vi "Autonomous Independent.vi"() -> ()   [LabVIEW 2016]
doc: "This VI is called when autonomous begins, and will automatically be terminated when autonomous ends. You can carry out timed or sensor driven robot movement independently without needing to return to the caller."
uses:
  <vilib>/Rock Robotics/WPI/Solenoid/WPI_SolenoidValue.ctl
  <vilib>/Rock Robotics/WPI/ThirdParty/Sensors/navX/_TypeDefs/FRIC_navX_DeviceNumbersTypeDef.ctl
  <vilib>/Rock Robotics/WPI/Utilities/WPI_GetSetVariantRefNum.vi
  <vilib>/Rock Robotics/Network Tables/NT Read String.vi
  <vilib>/Rock Robotics/WPI/Solenoid/WPI_SolenoidSetEnum.vi
  <vilib>/Rock Robotics/Network Tables/NT Write Number.vi
  <vilib>/addons/control/pid/pid.llb/PID (DBL).vi
  <vilib>/Rock Robotics/Network Tables/NT Write Numeric Array.vi
  <vilib>/addons/control/pid/NI_PID_pid.lvlib
panel:
  out "Distance 11":dbl
  out "Distance 10":dbl
  out "Distance 9":dbl
  out "Distance 8":dbl
  out "Distance 7":dbl
  out "Distance 6":dbl
  out "Distance 5":dbl
  out "Distance 4":dbl
  out "Distance 3":dbl
  out "Distance 2":dbl
  out "Distance 0":dbl
  out "Distance 1":dbl
  # "Be sure to right-click and choose Data Operations>>Make Current Value default if you want to save the array values with the VI"
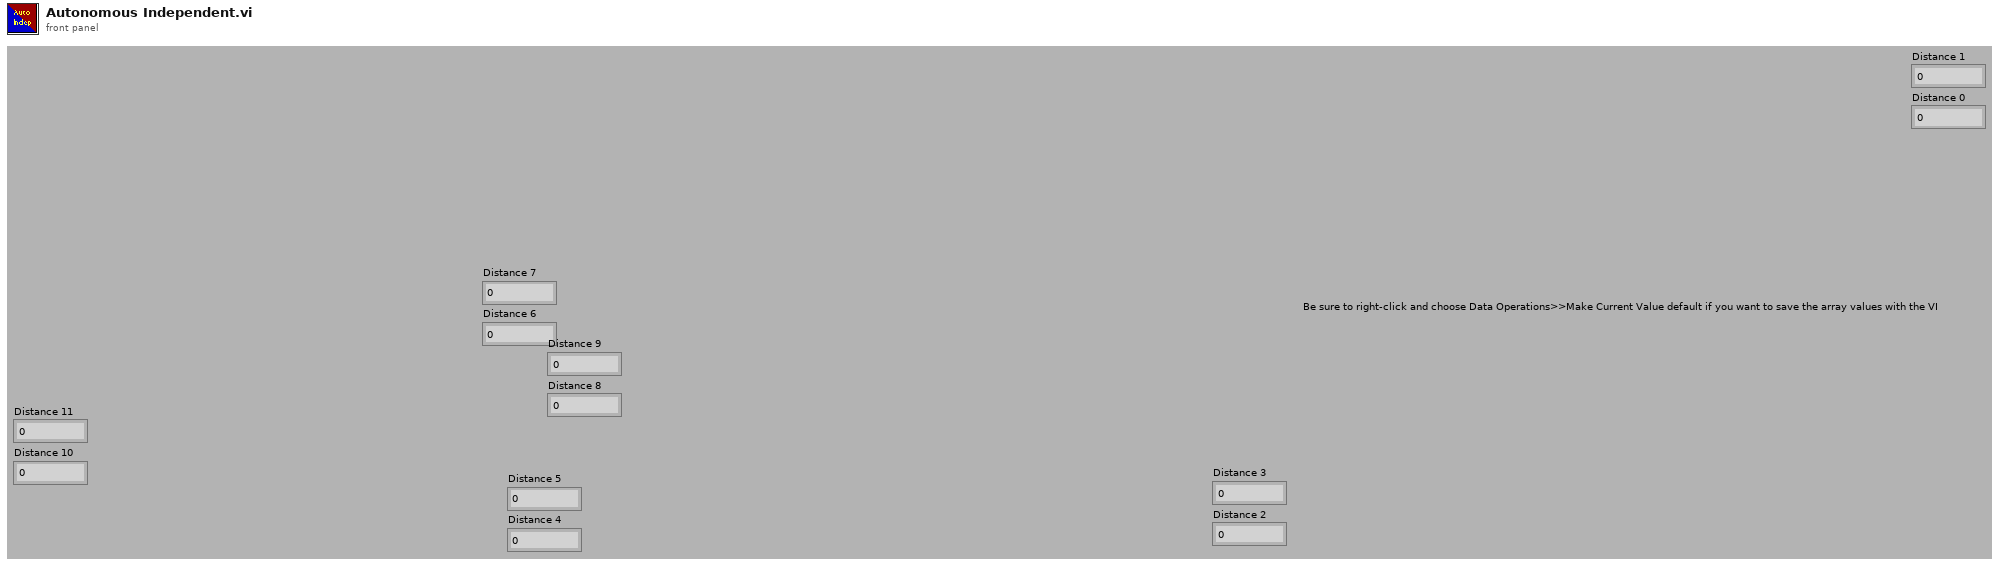
[diagram p1: front panel]
types:
  T1 = typedef "WPI_JoystickDevRef.ctl" = cluster{"Device":T2}
  T2 = typedef "WPI_JoystickDeviceEnum.ctl" = enum16{"USB 0", "USB 1", "USB 2", "USB 3", "USB 4", "USB 5"}
  T3 = typedef "WPI_SolenoidValue.ctl" = enum16{"Off", "On", "Forward", "Reverse"}
  T4 = typedef "FRIC_navX_DeviceNumbersTypeDef.ctl" = enum16{"Dev0", "Dev1", "Dev2", "Dev3"}
  T5 = cluster{"proportional gain (Kc)":dbl, "integral time (Ti, min)":dbl, "derivative time (Td, min)":dbl}
  T6 = typedef "WPI_SolenoidDevRef.ctl" = cluster{"DevStatus":errorcluster, "Pneumatics Control Module":u8, "Forward Solenoid Channel":T7, "Reverse Solenoid Channel":T7}
  T7 = typedef "WPI_SolenoidChannel.ctl" = enum8{"Solenoid 0", "Solenoid 1", "Solenoid 2", "Solenoid 3", "Solenoid 4", "Solenoid 5", "Solenoid 6", "Solenoid 7", "Invalid"}
  T8 = typedef "WPI_RobotDriveDevRef.ctl" = cluster{"DevStatus":errorcluster, "Motors[]":T9[], "Square Inputs":bool, "Max Output":dbl}
  T9 = typedef "WPI_MotorControlDeviceRef.ctl" = cluster{"DeviceStatus":errorcluster, "Type":T10, "PWM":cluster{"PWM Channel":T11, "DeadBand":T12}, "CAN":cluster{"Device Number":u8, "SetOutput VI Ref":variant, "GetOutput VI Ref":variant, "Enable VI Ref":variant, "Disable VI Ref":variant, "Data":variant}, "Invert":bool}
  T10 = typedef "WPI_MotorControlType.ctl" = enum16{"PWM", "CAN"}
  T11 = typedef "FPGA_DIOPWMChannel.ctl" = enum8{"PWM 0", "PWM 1", "PWM 2", "PWM 3", "PWM 4", "PWM 5", "PWM 6", "PWM 7", "PWM 8", "PWM 9", "PWM MXP 0", "PWM MXP 1", "PWM MXP 2", "PWM MXP 3", "PWM MXP 4", "PWM MXP 5", "PWM MXP 6", "PWM MXP 7", "PWM MXP 8", "PWM MXP 9", "Invalid"}
  T12 = typedef "WPI_PWMDeadband.ctl" = cluster{"Name":string, "maxPositivePwm":i32, "minPositivePwm":i32, "centerPwm":i32, "maxNegativePwm":i32, "minNegativePwm":i32, "angularRange":u16}
  T13 = typedef "WPI_EncoderDevRef.ctl" = cluster{"DevStatus":errorcluster, "EncoderIndex":T14, "CounterIndex":T15, "DistancePerCount":dbl, "Decoding Type":T16}
  T14 = typedef "FPGA_EncoderIdx.ctl" = enum8{"Enc 0", "Enc 1", "Enc 2", "Enc 3", "Enc 4", "Enc 5", "Enc 6", "Enc 7", "Invalid"}
  T15 = typedef "FPGA_CounterCtrSystemIndex.ctl" = enum8{"Ctr 0", "Ctr 1", "Ctr 2", "Ctr 3", "Ctr 4", "Ctr 5", "Ctr 6", "Ctr 7", "Invalid"}
  T16 = typedef "WPI_EncoderType.ctl" = enum16{"1x", "2x", "4x"}
  T17 = cluster{"Yaw":dbl, "Roll":dbl, "Pitch":dbl, "Heading":dbl, "Fused Heading":dbl}
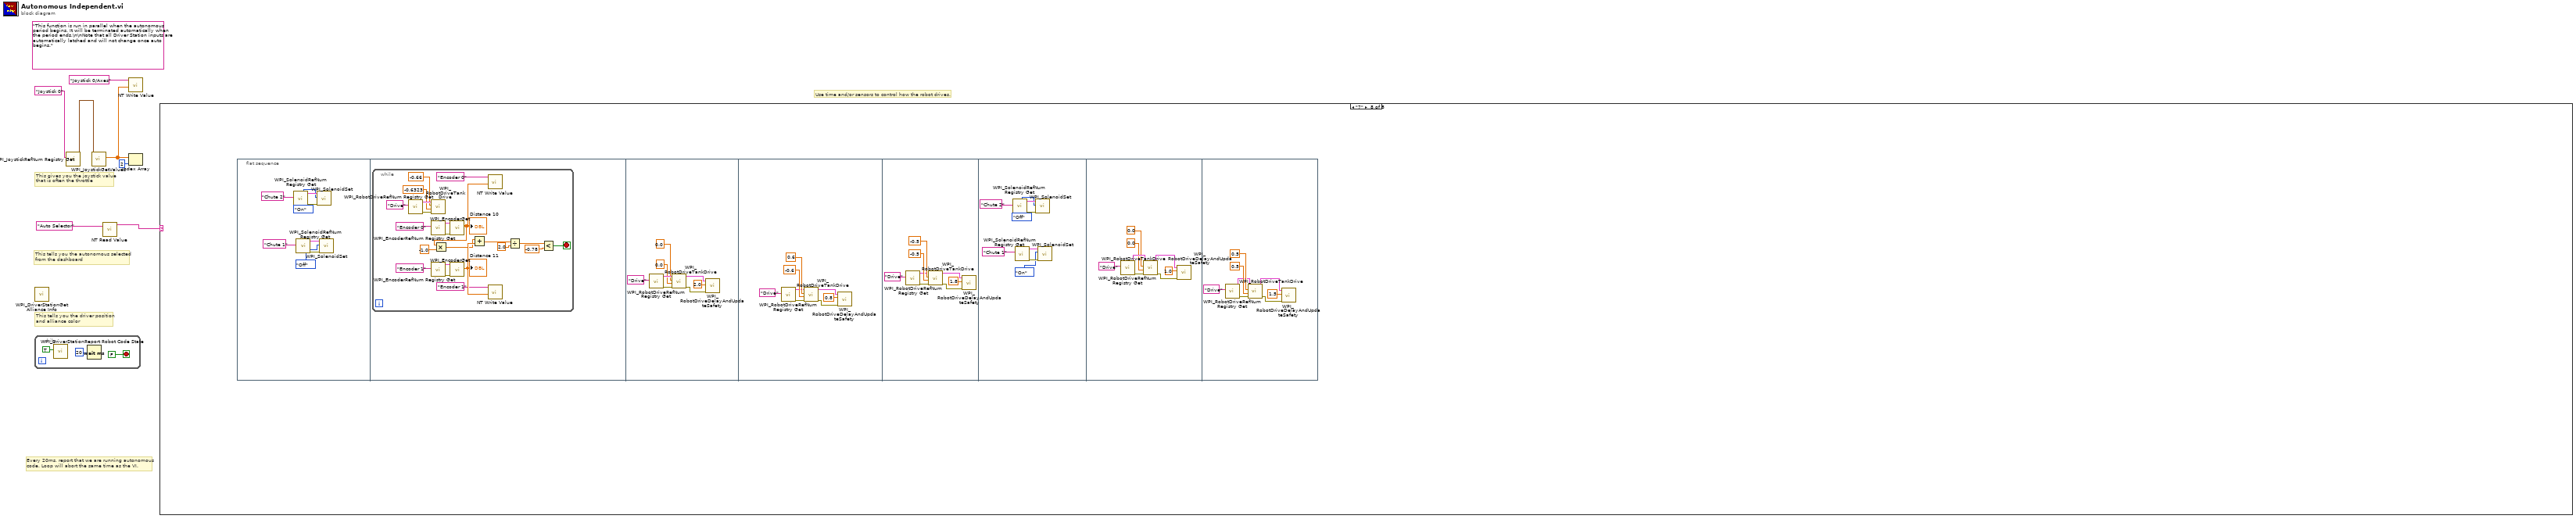
[diagram p0: block diagram]
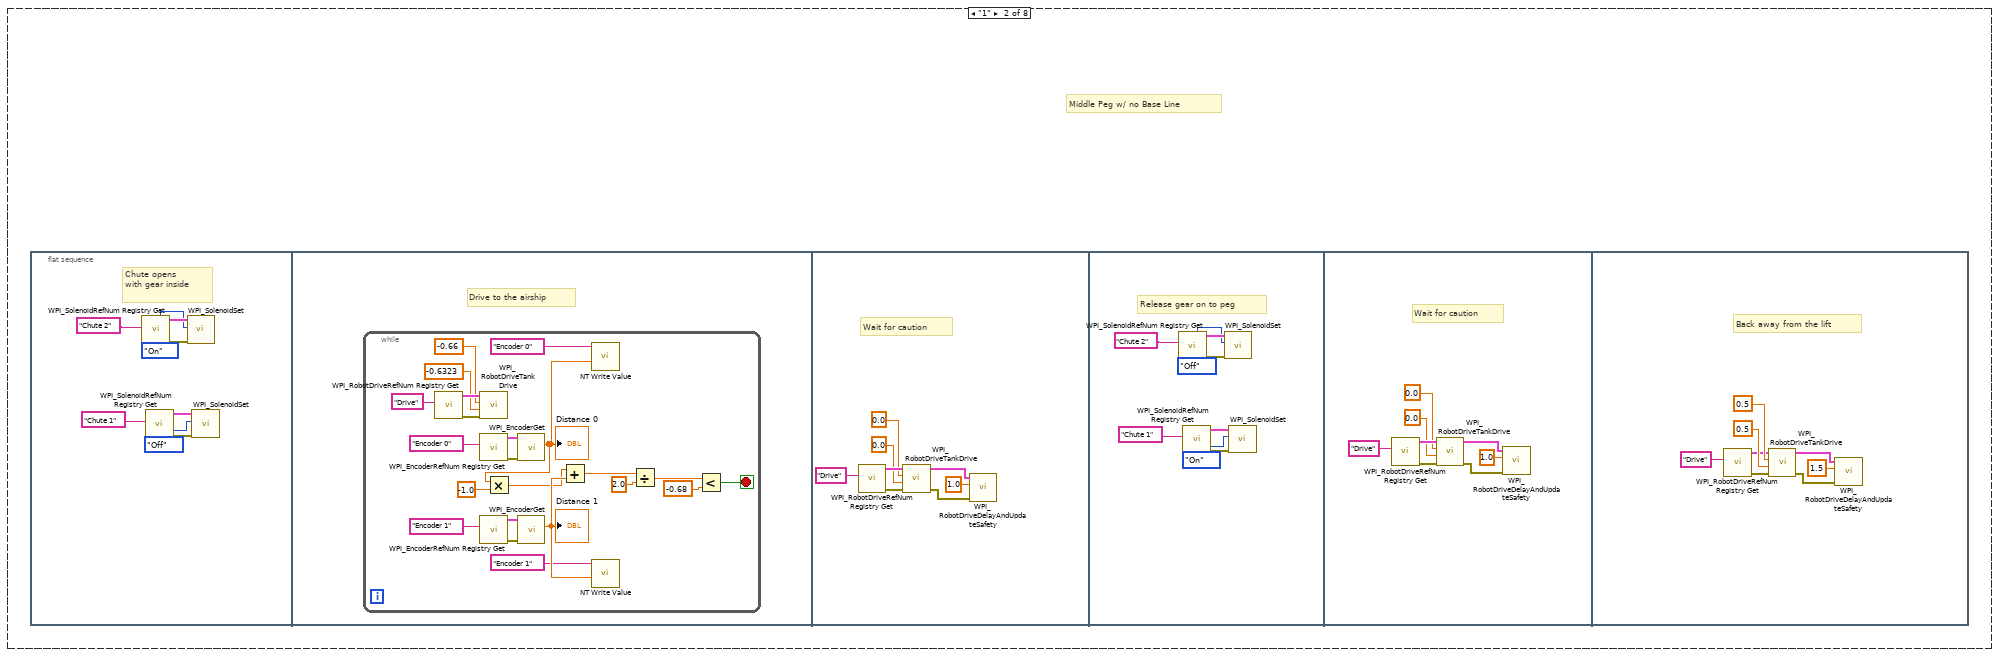
[diagram p3: hidden frame]
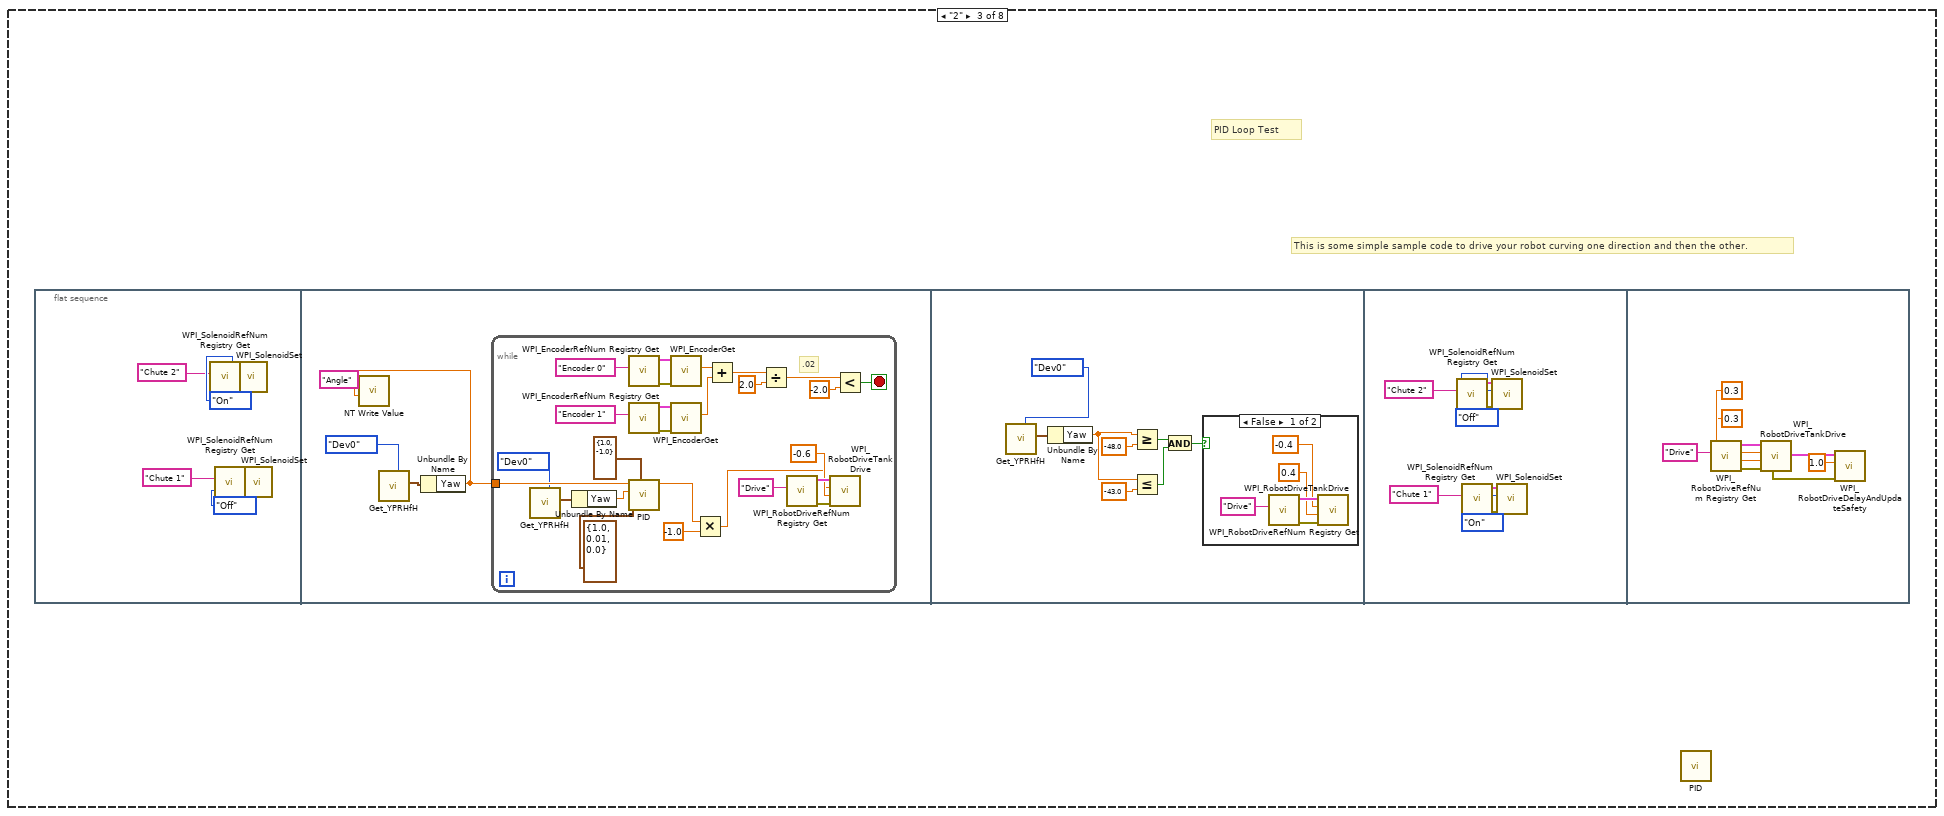
[diagram p4: hidden frame]
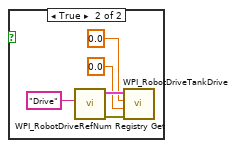
[diagram p5: hidden frame]
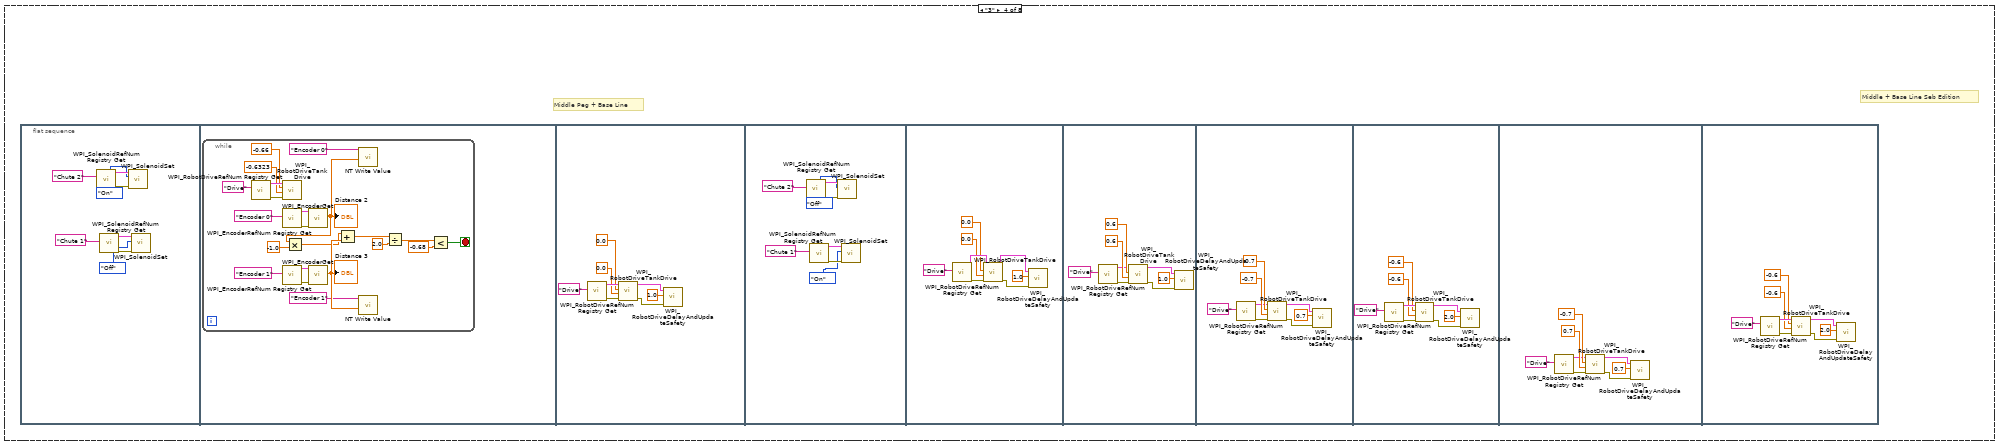
[diagram p6: hidden frame]
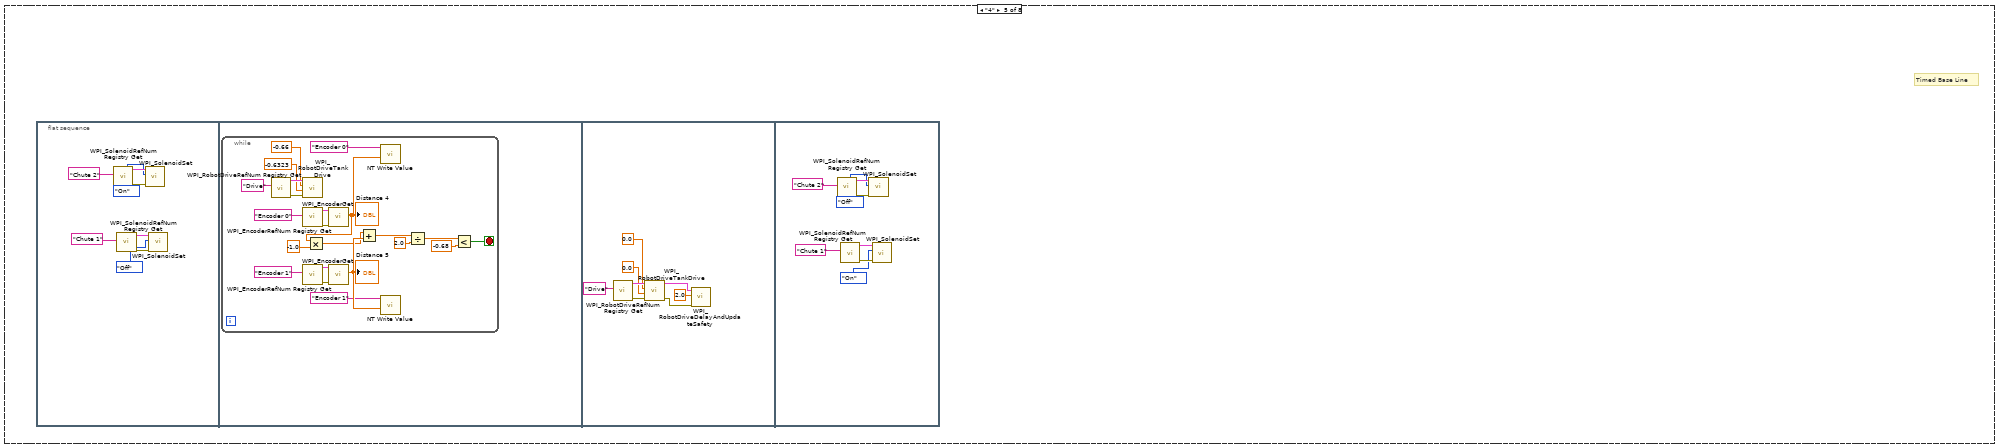
[diagram p7: hidden frame]
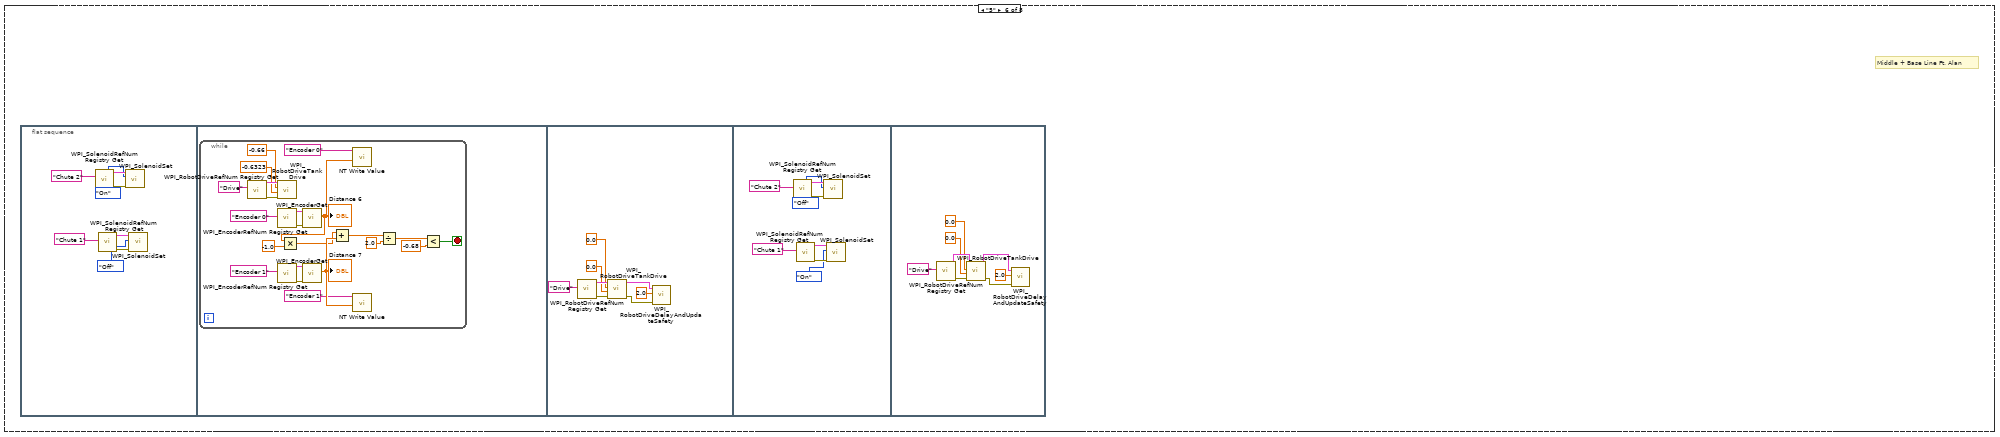
[diagram p8: hidden frame]
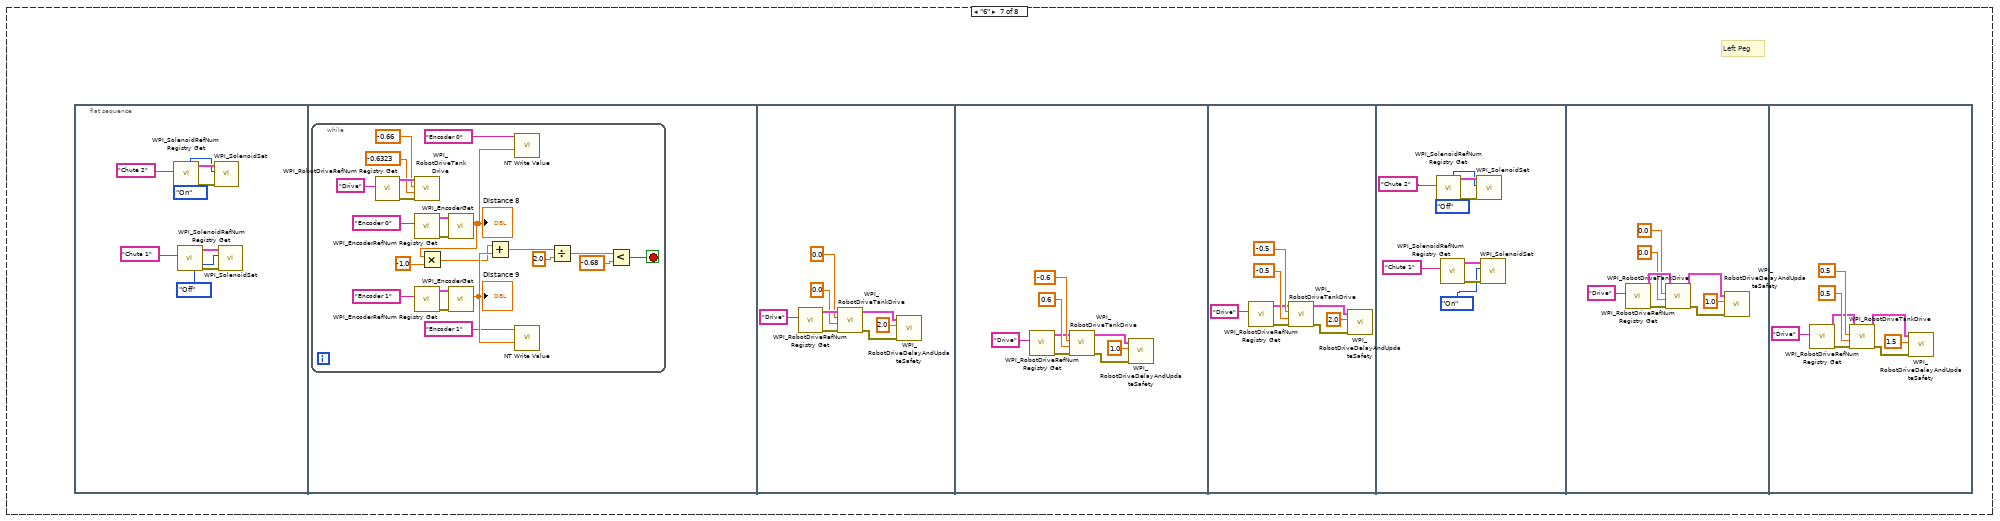
[diagram p9: hidden frame]
diagram:
  (unwired) "This function is run in parallel when the autonomous period begins. It will be terminated automatically when the period ends.\n\nNote that all Driver Station inputs are automatically latched and will not change once auto begins."
  # "This tells you the autonomous selected\nfrom the dashboard"
  # "Every 20ms, report that we are running autonomous\ncode. Loop will abort the same time as the VI."
  # "This gives you the joystick value\nthat is often the throttle"
  # "Use time and/or sensors to control how the robot drives."
  # "This tells you the driver position\nand alliance color"
  n1 = while {
    stop <- FALSE stop-if-true
    n2 = call <vilib>:"WPI_DriverStationReport Robot Code State.vi"("Autonomous"=TRUE) -> ()  [unwired: 10 in, 1 out]
    n3 = Wait (ms)(milliseconds to wait=u32 20) -> ()  [unwired: 1 out]
  }
  n4 = call <vilib>:"WPI_DriverStationGet Alliance Info.vi"() -> ()  [unwired: 12 out]
  n5 = call <vilib>:"WPI_JoystickRefNum Registry Get.vi"("refnum name"="Joystick 0") -> ("JoystickDevRef"=w6:T1)  [unwired: 1 in, 9 out]
  n6 = call <vilib>:"WPI_JoystickGetValues.vi"("JoystickDevRef"=w6) -> ("Axes"=w2:dbl[])  [unwired: 6 in, 4 out]
  n7 = call-poly <vilib>:"NT Read Value.vi"("Name"="Auto Selector") -> ("String"=w3:string)  [unwired: 9 in, 1 out]
  n8 = call-poly <vilib>:"NT Write Value.vi"("Numeric Array"=w2, "Name"="Joystick 0/Axes") -> ()  [unwired: 9 in, 1 out]
  n9 = Index Array(array=w2, index=2) -> ()  [unwired: 1 out]
  n10 = case shown="\"7\"" w3 {
    frame Default {
    }
    frame "1" {
      # "Middle Peg w/ no Base Line"
      n11 = flat-sequence {
        frame #0 {
          # "Chute opens\nwith gear inside"
          n12 = call <vilib>:"WPI_SolenoidRefNum Registry Get.vi"("refnum name"="Chute 2") -> ("error out"=w18:errorcluster, "SolenoidDevRef"=w17:T6)  [unwired: 9 in]
          n13 = call <vilib>:"WPI_SolenoidRefNum Registry Get.vi"("refnum name"="Chute 1") -> ("error out"=w14:errorcluster, "SolenoidDevRef"=w13:T6)  [unwired: 9 in]
          n14 = call-poly <vilib>:"WPI_SolenoidSet.vi"("error in (no error)"=w18, "Value"=WPI_SolenoidValue."On", "SolenoidDevRef"=w17) -> ()  [unwired: 7 in, 2 out]
          n15 = call-poly <vilib>:"WPI_SolenoidSet.vi"("error in (no error)"=w14, "Value"=WPI_SolenoidValue."Off", "SolenoidDevRef"=w13) -> ()  [unwired: 7 in, 2 out]
        }
        frame #1 {
          # "Drive to the airship"
          n16 = while {
            stop <- w26 stop-if-true
            n17 = call <vilib>:"WPI_RobotDriveRefNum Registry Get.vi"("refnum name"="Drive") -> ("error out"=w39:errorcluster, "RobotDriveDevRef"=w40:T8)  [unwired: 9 in]
            n18 = call <vilib>:"WPI_RobotDriveTankDrive.vi"("error in (no error)"=w39, "Right axis value"=-0.6323, "Left axis value"=-0.66, "RobotDriveDevRef"=w40) -> ()  [unwired: 5 in, 3 out]
            n19 = call <vilib>:"WPI_EncoderRefNum Registry Get.vi"("refnum name"="Encoder 0") -> ("error out"=w35:errorcluster, "EncoderDevRef"=w34:T13)  [unwired: 9 in]
            n20 = call <vilib>:"WPI_EncoderRefNum Registry Get.vi"("refnum name"="Encoder 1") -> ("error out"=w32:errorcluster, "EncoderDevRef"=w31:T13)  [unwired: 9 in]
            n21 = call <vilib>:"WPI_EncoderGet.vi"("error in (no error)"=w35, "EncoderDevRef"=w34) -> ("Distance"=w20:dbl)  [unwired: 4 in, 5 out]
            "Distance 0" <- w20
            n22 = Multiply(x=w20, y=-1.0) -> (x*y=w19:dbl)
            n23 = call <vilib>:"WPI_EncoderGet.vi"("error in (no error)"=w32, "EncoderDevRef"=w31) -> ("Distance"=w23:dbl)  [unwired: 4 in, 5 out]
            "Distance 1" <- w23
            n24 = Add(x=w19, y=w23) -> (x+y=w29:dbl)
            n25 = call-poly <vilib>:"NT Write Value.vi"("Numeric"=w20, "Name"="Encoder 0") -> ()  [unwired: 9 in, 1 out]
            n26 = call-poly <vilib>:"NT Write Value.vi"("Numeric"=w23, "Name"="Encoder 1") -> ()  [unwired: 9 in, 1 out]
            n27 = Divide(x=w29, y=2.0) -> (x/y=w27:dbl)
            n28 = Less?(x=w27, y=-0.68) -> (x < y?=w26:bool)
          }
        }
        frame #2 {
          # "Wait for caution"
          n29 = call <vilib>:"WPI_RobotDriveRefNum Registry Get.vi"("refnum name"="Drive") -> ("error out"=w44:errorcluster, "RobotDriveDevRef"=w45:T8)  [unwired: 9 in]
          n30 = call <vilib>:"WPI_RobotDriveTankDrive.vi"("error in (no error)"=w44, "Right axis value"=0.0, "Left axis value"=0.0, "RobotDriveDevRef"=w45) -> ("error out"=w47:errorcluster, "RobotDriveDevRef"=w46:T8)  [unwired: 5 in, 1 out]
          n31 = call <vilib>:"WPI_RobotDriveDelayAndUpdateSafety.vi"("error in (no error)"=w47, "Delay (s)"=1.0, "RobotDriveDevRef"=w46) -> ()  [unwired: 7 in, 2 out]
        }
        frame #3 {
          # "Release gear on to peg"
          n32 = call <vilib>:"WPI_SolenoidRefNum Registry Get.vi"("refnum name"="Chute 2") -> ("error out"=w56:errorcluster, "SolenoidDevRef"=w55:T6)  [unwired: 9 in]
          n33 = call <vilib>:"WPI_SolenoidRefNum Registry Get.vi"("refnum name"="Chute 1") -> ("error out"=w52:errorcluster, "SolenoidDevRef"=w51:T6)  [unwired: 9 in]
          n34 = call-poly <vilib>:"WPI_SolenoidSet.vi"("error in (no error)"=w56, "Value"=WPI_SolenoidValue."Off", "SolenoidDevRef"=w55) -> ()  [unwired: 7 in, 2 out]
          n35 = call-poly <vilib>:"WPI_SolenoidSet.vi"("error in (no error)"=w52, "Value"=WPI_SolenoidValue."On", "SolenoidDevRef"=w51) -> ()  [unwired: 7 in, 2 out]
        }
        frame #4 {
          # "Wait for caution"
          n36 = call <vilib>:"WPI_RobotDriveRefNum Registry Get.vi"("refnum name"="Drive") -> ("error out"=w60:errorcluster, "RobotDriveDevRef"=w61:T8)  [unwired: 9 in]
          n37 = call <vilib>:"WPI_RobotDriveTankDrive.vi"("error in (no error)"=w60, "Right axis value"=0.0, "Left axis value"=0.0, "RobotDriveDevRef"=w61) -> ("error out"=w63:errorcluster, "RobotDriveDevRef"=w62:T8)  [unwired: 5 in, 1 out]
          n38 = call <vilib>:"WPI_RobotDriveDelayAndUpdateSafety.vi"("error in (no error)"=w63, "Delay (s)"=1.0, "RobotDriveDevRef"=w62) -> ()  [unwired: 7 in, 2 out]
        }
        frame #5 {
          # "Back away from the lift"
          n39 = call <vilib>:"WPI_RobotDriveRefNum Registry Get.vi"("refnum name"="Drive") -> ("error out"=w69:errorcluster, "RobotDriveDevRef"=w68:T8)  [unwired: 9 in]
          n40 = call <vilib>:"WPI_RobotDriveTankDrive.vi"("error in (no error)"=w69, "Right axis value"=0.5, "Left axis value"=0.5, "RobotDriveDevRef"=w68) -> ("error out"=w66:errorcluster, "RobotDriveDevRef"=w67:T8)  [unwired: 5 in, 1 out]
          n41 = call <vilib>:"WPI_RobotDriveDelayAndUpdateSafety.vi"("error in (no error)"=w66, "Delay (s)"=1.5, "RobotDriveDevRef"=w67) -> ()  [unwired: 7 in, 2 out]
        }
      }
    }
    frame "2" {
      # "PID Loop Test"
      # "This is some simple sample code to drive your robot curving one direction and then the other."
      n42 = flat-sequence {
        frame #0 {
          n43 = call <vilib>:"WPI_SolenoidRefNum Registry Get.vi"("refnum name"="Chute 2") -> ("error out"=w80:errorcluster, "SolenoidDevRef"=w79:T6)  [unwired: 9 in]
          n44 = call <vilib>:"WPI_SolenoidRefNum Registry Get.vi"("refnum name"="Chute 1") -> ("error out"=w76:errorcluster, "SolenoidDevRef"=w75:T6)  [unwired: 9 in]
          n45 = call-poly <vilib>:"WPI_SolenoidSet.vi"("error in (no error)"=w80, "Value"=WPI_SolenoidValue."On", "SolenoidDevRef"=w79) -> ()  [unwired: 7 in, 2 out]
          n46 = call-poly <vilib>:"WPI_SolenoidSet.vi"("error in (no error)"=w76, "Value"=WPI_SolenoidValue."Off", "SolenoidDevRef"=w75) -> ()  [unwired: 7 in, 2 out]
        }
        frame #1 {
          n47 = call <vilib>:"Get_YPRHfH.vi"("Device Number"=FRIC_navX_DeviceNumbersTypeDef."Dev0") -> ("YRPHfH"=w84:T17)  [unwired: 10 in]
          n48 = Unbundle By Name(w84) -> ("Yaw"=w83:dbl)
          n49 = call-poly <vilib>:"NT Write Value.vi"("Numeric"=w83, "Name"="Angle") -> ()  [unwired: 9 in, 1 out]
          n50 = while {
            tunnel: w83 -> [w96]
            stop <- w99 stop-if-true
            # ".02"
            n51 = call <vilib>:"Get_YPRHfH.vi"("Device Number"=FRIC_navX_DeviceNumbersTypeDef."Dev0") -> ("YRPHfH"=w97:T17)  [unwired: 10 in]
            n52 = Unbundle By Name(w97) -> ("Yaw"=w95:dbl)
            n53 = call <vilib>:"WPI_EncoderRefNum Registry Get.vi"("refnum name"="Encoder 0") -> ("error out"=w110:errorcluster, "EncoderDevRef"=w109:T13)  [unwired: 9 in]
            n54 = call <vilib>:"WPI_EncoderRefNum Registry Get.vi"("refnum name"="Encoder 1") -> ("error out"=w107:errorcluster, "EncoderDevRef"=w106:T13)  [unwired: 9 in]
            n55 = call-poly <vilib>:"PID.vi"("output range"=cluster{"output high":dbl, "output low":dbl} {"output high"=1.0, "output low"=-1.0}, "PID gains"=T5 {"proportional gain (Kc)"=1.0, "integral time (Ti, min)"=0.01, "derivative time (Td, min)"=0.0}, "process variable"=w95, "setpoint"=w96) -> ("output"=w87:dbl)  [unwired: 6 in, 1 out]
            n56 = call <vilib>:"WPI_EncoderGet.vi"("error in (no error)"=w110, "EncoderDevRef"=w109) -> ("Distance"=w103:dbl)  [unwired: 4 in, 5 out]
            n57 = call <vilib>:"WPI_EncoderGet.vi"("error in (no error)"=w107, "EncoderDevRef"=w106) -> ("Distance"=w104:dbl)  [unwired: 4 in, 5 out]
            n58 = Multiply(x=w87, y=-1.0) -> (x*y=w86:dbl)
            n59 = Add(x=w103, y=w104) -> (x+y=w102:dbl)
            n60 = Divide(x=w102, y=2.0) -> (x/y=w100:dbl)
            n61 = call <vilib>:"WPI_RobotDriveRefNum Registry Get.vi"("refnum name"="Drive") -> ("error out"=w91:errorcluster, "RobotDriveDevRef"=w92:T8)  [unwired: 9 in]
            n62 = call <vilib>:"WPI_RobotDriveTankDrive.vi"("error in (no error)"=w91, "Right axis value"=-0.6, "Left axis value"=w86, "RobotDriveDevRef"=w92) -> ()  [unwired: 5 in, 3 out]
            n63 = Less?(x=w100, y=-2.0) -> (x < y?=w99:bool)
          }
        }
        frame #2 {
          n64 = call <vilib>:"Get_YPRHfH.vi"("Device Number"=FRIC_navX_DeviceNumbersTypeDef."Dev0") -> ("YRPHfH"=w118:T17)  [unwired: 10 in]
          n65 = Unbundle By Name(w118) -> ("Yaw"=w113:dbl)
          n66 = Greater Or Equal?(x=w113, y=-48.0) -> (x >= y?=w116:bool)
          n67 = Less Or Equal?(x=w113, y=-43.0) -> (x <= y?=w115:bool)
          n68 = And(x=w116, y=w115) -> (x .and. y?=w112:bool)
          n69 = case shown="False" w112 {
            frame False {
              n70 = call <vilib>:"WPI_RobotDriveRefNum Registry Get.vi"("refnum name"="Drive") -> ("error out"=w122:errorcluster, "RobotDriveDevRef"=w123:T8)  [unwired: 9 in]
              n71 = call <vilib>:"WPI_RobotDriveTankDrive.vi"("error in (no error)"=w122, "Right axis value"=0.4, "Left axis value"=-0.4, "RobotDriveDevRef"=w123) -> ()  [unwired: 5 in, 3 out]
            }
            frame True {
              n72 = call <vilib>:"WPI_RobotDriveRefNum Registry Get.vi"("refnum name"="Drive") -> ("error out"=w127:errorcluster, "RobotDriveDevRef"=w128:T8)  [unwired: 9 in]
              n73 = call <vilib>:"WPI_RobotDriveTankDrive.vi"("error in (no error)"=w127, "Right axis value"=0.0, "Left axis value"=0.0, "RobotDriveDevRef"=w128) -> ()  [unwired: 5 in, 3 out]
            }
          }
        }
        frame #3 {
          n74 = call <vilib>:"WPI_SolenoidRefNum Registry Get.vi"("refnum name"="Chute 2") -> ("error out"=w136:errorcluster, "SolenoidDevRef"=w135:T6)  [unwired: 9 in]
          n75 = call <vilib>:"WPI_SolenoidRefNum Registry Get.vi"("refnum name"="Chute 1") -> ("error out"=w132:errorcluster, "SolenoidDevRef"=w131:T6)  [unwired: 9 in]
          n76 = call-poly <vilib>:"WPI_SolenoidSet.vi"("error in (no error)"=w136, "Value"=WPI_SolenoidValue."Off", "SolenoidDevRef"=w135) -> ()  [unwired: 7 in, 2 out]
          n77 = call-poly <vilib>:"WPI_SolenoidSet.vi"("error in (no error)"=w132, "Value"=WPI_SolenoidValue."On", "SolenoidDevRef"=w131) -> ()  [unwired: 7 in, 2 out]
        }
        frame #4 {
          n78 = call <vilib>:"WPI_RobotDriveRefNum Registry Get.vi"("refnum name"="Drive") -> ("error out"=w141:errorcluster, "RobotDriveDevRef"=w140:T8)  [unwired: 9 in]
          n79 = call <vilib>:"WPI_RobotDriveTankDrive.vi"("error in (no error)"=w141, "Right axis value"=0.3, "Left axis value"=0.3, "RobotDriveDevRef"=w140) -> ("error out"=w138:errorcluster, "RobotDriveDevRef"=w139:T8)  [unwired: 5 in, 1 out]
          n80 = call <vilib>:"WPI_RobotDriveDelayAndUpdateSafety.vi"("error in (no error)"=w138, "Delay (s)"=1.0, "RobotDriveDevRef"=w139) -> ()  [unwired: 7 in, 2 out]
        }
      }
      n81 = call-poly <vilib>:"PID.vi"() -> ()  [unwired: 10 in, 2 out]
    }
    frame "3" {
      # "Middle + Base Line Seb Edition"
      # "Middle Peg + Base Line"
      n82 = flat-sequence {
        frame #0 {
          n83 = call <vilib>:"WPI_SolenoidRefNum Registry Get.vi"("refnum name"="Chute 2") -> ("error out"=w152:errorcluster, "SolenoidDevRef"=w151:T6)  [unwired: 9 in]
          n84 = call <vilib>:"WPI_SolenoidRefNum Registry Get.vi"("refnum name"="Chute 1") -> ("error out"=w148:errorcluster, "SolenoidDevRef"=w147:T6)  [unwired: 9 in]
          n85 = call-poly <vilib>:"WPI_SolenoidSet.vi"("error in (no error)"=w152, "Value"=WPI_SolenoidValue."On", "SolenoidDevRef"=w151) -> ()  [unwired: 7 in, 2 out]
          n86 = call-poly <vilib>:"WPI_SolenoidSet.vi"("error in (no error)"=w148, "Value"=WPI_SolenoidValue."Off", "SolenoidDevRef"=w147) -> ()  [unwired: 7 in, 2 out]
        }
        frame #1 {
          n87 = while {
            stop <- w160 stop-if-true
            n88 = call <vilib>:"WPI_RobotDriveRefNum Registry Get.vi"("refnum name"="Drive") -> ("error out"=w173:errorcluster, "RobotDriveDevRef"=w174:T8)  [unwired: 9 in]
            n89 = call <vilib>:"WPI_RobotDriveTankDrive.vi"("error in (no error)"=w173, "Right axis value"=-0.6323, "Left axis value"=-0.66, "RobotDriveDevRef"=w174) -> ()  [unwired: 5 in, 3 out]
            n90 = call <vilib>:"WPI_EncoderRefNum Registry Get.vi"("refnum name"="Encoder 0") -> ("error out"=w169:errorcluster, "EncoderDevRef"=w168:T13)  [unwired: 9 in]
            n91 = call <vilib>:"WPI_EncoderRefNum Registry Get.vi"("refnum name"="Encoder 1") -> ("error out"=w166:errorcluster, "EncoderDevRef"=w165:T13)  [unwired: 9 in]
            n92 = call <vilib>:"WPI_EncoderGet.vi"("error in (no error)"=w169, "EncoderDevRef"=w168) -> ("Distance"=w154:dbl)  [unwired: 4 in, 5 out]
            "Distance 2" <- w154
            n93 = Multiply(x=w154, y=-1.0) -> (x*y=w153:dbl)
            n94 = call <vilib>:"WPI_EncoderGet.vi"("error in (no error)"=w166, "EncoderDevRef"=w165) -> ("Distance"=w157:dbl)  [unwired: 4 in, 5 out]
            "Distance 3" <- w157
            n95 = Add(x=w153, y=w157) -> (x+y=w163:dbl)
            n96 = call-poly <vilib>:"NT Write Value.vi"("Numeric"=w154, "Name"="Encoder 0") -> ()  [unwired: 9 in, 1 out]
            n97 = call-poly <vilib>:"NT Write Value.vi"("Numeric"=w157, "Name"="Encoder 1") -> ()  [unwired: 9 in, 1 out]
            n98 = Divide(x=w163, y=2.0) -> (x/y=w161:dbl)
            n99 = Less?(x=w161, y=-0.68) -> (x < y?=w160:bool)
          }
        }
        frame #2 {
          n100 = call <vilib>:"WPI_RobotDriveRefNum Registry Get.vi"("refnum name"="Drive") -> ("error out"=w178:errorcluster, "RobotDriveDevRef"=w179:T8)  [unwired: 9 in]
          n101 = call <vilib>:"WPI_RobotDriveTankDrive.vi"("error in (no error)"=w178, "Right axis value"=0.0, "Left axis value"=0.0, "RobotDriveDevRef"=w179) -> ("error out"=w181:errorcluster, "RobotDriveDevRef"=w180:T8)  [unwired: 5 in, 1 out]
          n102 = call <vilib>:"WPI_RobotDriveDelayAndUpdateSafety.vi"("error in (no error)"=w181, "Delay (s)"=1.0, "RobotDriveDevRef"=w180) -> ()  [unwired: 7 in, 2 out]
        }
        frame #3 {
          n103 = call <vilib>:"WPI_SolenoidRefNum Registry Get.vi"("refnum name"="Chute 2") -> ("error out"=w190:errorcluster, "SolenoidDevRef"=w189:T6)  [unwired: 9 in]
          n104 = call <vilib>:"WPI_SolenoidRefNum Registry Get.vi"("refnum name"="Chute 1") -> ("error out"=w186:errorcluster, "SolenoidDevRef"=w185:T6)  [unwired: 9 in]
          n105 = call-poly <vilib>:"WPI_SolenoidSet.vi"("error in (no error)"=w190, "Value"=WPI_SolenoidValue."Off", "SolenoidDevRef"=w189) -> ()  [unwired: 7 in, 2 out]
          n106 = call-poly <vilib>:"WPI_SolenoidSet.vi"("error in (no error)"=w186, "Value"=WPI_SolenoidValue."On", "SolenoidDevRef"=w185) -> ()  [unwired: 7 in, 2 out]
        }
        frame #4 {
          n107 = call <vilib>:"WPI_RobotDriveRefNum Registry Get.vi"("refnum name"="Drive") -> ("error out"=w194:errorcluster, "RobotDriveDevRef"=w195:T8)  [unwired: 9 in]
          n108 = call <vilib>:"WPI_RobotDriveTankDrive.vi"("error in (no error)"=w194, "Right axis value"=0.0, "Left axis value"=0.0, "RobotDriveDevRef"=w195) -> ("error out"=w197:errorcluster, "RobotDriveDevRef"=w196:T8)  [unwired: 5 in, 1 out]
          n109 = call <vilib>:"WPI_RobotDriveDelayAndUpdateSafety.vi"("error in (no error)"=w197, "Delay (s)"=1.0, "RobotDriveDevRef"=w196) -> ()  [unwired: 7 in, 2 out]
        }
        frame #5 {
          n110 = call <vilib>:"WPI_RobotDriveRefNum Registry Get.vi"("refnum name"="Drive") -> ("error out"=w203:errorcluster, "RobotDriveDevRef"=w202:T8)  [unwired: 9 in]
          n111 = call <vilib>:"WPI_RobotDriveTankDrive.vi"("error in (no error)"=w203, "Right axis value"=0.6, "Left axis value"=0.6, "RobotDriveDevRef"=w202) -> ("error out"=w200:errorcluster, "RobotDriveDevRef"=w201:T8)  [unwired: 5 in, 1 out]
          n112 = call <vilib>:"WPI_RobotDriveDelayAndUpdateSafety.vi"("error in (no error)"=w200, "Delay (s)"=1.0, "RobotDriveDevRef"=w201) -> ()  [unwired: 7 in, 2 out]
        }
        frame #6 {
          n113 = call <vilib>:"WPI_RobotDriveRefNum Registry Get.vi"("refnum name"="Drive") -> ("error out"=w211:errorcluster, "RobotDriveDevRef"=w210:T8)  [unwired: 9 in]
          n114 = call <vilib>:"WPI_RobotDriveTankDrive.vi"("error in (no error)"=w211, "Right axis value"=-0.7, "Left axis value"=0.7, "RobotDriveDevRef"=w210) -> ("error out"=w208:errorcluster, "RobotDriveDevRef"=w209:T8)  [unwired: 5 in, 1 out]
          n115 = call <vilib>:"WPI_RobotDriveDelayAndUpdateSafety.vi"("error in (no error)"=w208, "Delay (s)"=0.7, "RobotDriveDevRef"=w209) -> ()  [unwired: 7 in, 2 out]
        }
        frame #7 {
          n116 = call <vilib>:"WPI_RobotDriveRefNum Registry Get.vi"("refnum name"="Drive") -> ("error out"=w218:errorcluster, "RobotDriveDevRef"=w219:T8)  [unwired: 9 in]
          n117 = call <vilib>:"WPI_RobotDriveTankDrive.vi"("error in (no error)"=w218, "Right axis value"=-0.6, "Left axis value"=-0.6, "RobotDriveDevRef"=w219) -> ("error out"=w221:errorcluster, "RobotDriveDevRef"=w220:T8)  [unwired: 5 in, 1 out]
          n118 = call <vilib>:"WPI_RobotDriveDelayAndUpdateSafety.vi"("error in (no error)"=w221, "Delay (s)"=2.0, "RobotDriveDevRef"=w220) -> ()  [unwired: 7 in, 2 out]
        }
        frame #8 {
          n119 = call <vilib>:"WPI_RobotDriveRefNum Registry Get.vi"("refnum name"="Drive") -> ("error out"=w227:errorcluster, "RobotDriveDevRef"=w226:T8)  [unwired: 9 in]
          n120 = call <vilib>:"WPI_RobotDriveTankDrive.vi"("error in (no error)"=w227, "Right axis value"=0.7, "Left axis value"=-0.7, "RobotDriveDevRef"=w226) -> ("error out"=w224:errorcluster, "RobotDriveDevRef"=w225:T8)  [unwired: 5 in, 1 out]
          n121 = call <vilib>:"WPI_RobotDriveDelayAndUpdateSafety.vi"("error in (no error)"=w224, "Delay (s)"=0.7, "RobotDriveDevRef"=w225) -> ()  [unwired: 7 in, 2 out]
        }
        frame #9 {
          n122 = call <vilib>:"WPI_RobotDriveRefNum Registry Get.vi"("refnum name"="Drive") -> ("error out"=w234:errorcluster, "RobotDriveDevRef"=w235:T8)  [unwired: 9 in]
          n123 = call <vilib>:"WPI_RobotDriveTankDrive.vi"("error in (no error)"=w234, "Right axis value"=-0.6, "Left axis value"=-0.6, "RobotDriveDevRef"=w235) -> ("error out"=w237:errorcluster, "RobotDriveDevRef"=w236:T8)  [unwired: 5 in, 1 out]
          n124 = call <vilib>:"WPI_RobotDriveDelayAndUpdateSafety.vi"("error in (no error)"=w237, "Delay (s)"=2.0, "RobotDriveDevRef"=w236) -> ()  [unwired: 7 in, 2 out]
        }
      }
    }
    frame "4" {
      # "Timed Base Line"
      n125 = flat-sequence {
        frame #0 {
          n126 = call <vilib>:"WPI_SolenoidRefNum Registry Get.vi"("refnum name"="Chute 2") -> ("error out"=w246:errorcluster, "SolenoidDevRef"=w245:T6)  [unwired: 9 in]
          n127 = call <vilib>:"WPI_SolenoidRefNum Registry Get.vi"("refnum name"="Chute 1") -> ("error out"=w242:errorcluster, "SolenoidDevRef"=w241:T6)  [unwired: 9 in]
          n128 = call-poly <vilib>:"WPI_SolenoidSet.vi"("error in (no error)"=w246, "Value"=WPI_SolenoidValue."On", "SolenoidDevRef"=w245) -> ()  [unwired: 7 in, 2 out]
          n129 = call-poly <vilib>:"WPI_SolenoidSet.vi"("error in (no error)"=w242, "Value"=WPI_SolenoidValue."Off", "SolenoidDevRef"=w241) -> ()  [unwired: 7 in, 2 out]
        }
        frame #1 {
          n130 = while {
            stop <- w254 stop-if-true
            n131 = call <vilib>:"WPI_RobotDriveRefNum Registry Get.vi"("refnum name"="Drive") -> ("error out"=w267:errorcluster, "RobotDriveDevRef"=w268:T8)  [unwired: 9 in]
            n132 = call <vilib>:"WPI_RobotDriveTankDrive.vi"("error in (no error)"=w267, "Right axis value"=-0.6323, "Left axis value"=-0.66, "RobotDriveDevRef"=w268) -> ()  [unwired: 5 in, 3 out]
            n133 = call <vilib>:"WPI_EncoderRefNum Registry Get.vi"("refnum name"="Encoder 0") -> ("error out"=w263:errorcluster, "EncoderDevRef"=w262:T13)  [unwired: 9 in]
            n134 = call <vilib>:"WPI_EncoderRefNum Registry Get.vi"("refnum name"="Encoder 1") -> ("error out"=w260:errorcluster, "EncoderDevRef"=w259:T13)  [unwired: 9 in]
            n135 = call <vilib>:"WPI_EncoderGet.vi"("error in (no error)"=w263, "EncoderDevRef"=w262) -> ("Distance"=w248:dbl)  [unwired: 4 in, 5 out]
            "Distance 4" <- w248
            n136 = Multiply(x=w248, y=-1.0) -> (x*y=w247:dbl)
            n137 = call <vilib>:"WPI_EncoderGet.vi"("error in (no error)"=w260, "EncoderDevRef"=w259) -> ("Distance"=w251:dbl)  [unwired: 4 in, 5 out]
            "Distance 5" <- w251
            n138 = Add(x=w247, y=w251) -> (x+y=w257:dbl)
            n139 = call-poly <vilib>:"NT Write Value.vi"("Numeric"=w248, "Name"="Encoder 0") -> ()  [unwired: 9 in, 1 out]
            n140 = call-poly <vilib>:"NT Write Value.vi"("Numeric"=w251, "Name"="Encoder 1") -> ()  [unwired: 9 in, 1 out]
            n141 = Divide(x=w257, y=2.0) -> (x/y=w255:dbl)
            n142 = Less?(x=w255, y=-0.68) -> (x < y?=w254:bool)
          }
        }
        frame #2 {
          n143 = call <vilib>:"WPI_RobotDriveRefNum Registry Get.vi"("refnum name"="Drive") -> ("error out"=w272:errorcluster, "RobotDriveDevRef"=w273:T8)  [unwired: 9 in]
          n144 = call <vilib>:"WPI_RobotDriveTankDrive.vi"("error in (no error)"=w272, "Right axis value"=0.0, "Left axis value"=0.0, "RobotDriveDevRef"=w273) -> ("error out"=w275:errorcluster, "RobotDriveDevRef"=w274:T8)  [unwired: 5 in, 1 out]
          n145 = call <vilib>:"WPI_RobotDriveDelayAndUpdateSafety.vi"("error in (no error)"=w275, "Delay (s)"=2.0, "RobotDriveDevRef"=w274) -> ()  [unwired: 7 in, 2 out]
        }
        frame #3 {
          n146 = call <vilib>:"WPI_SolenoidRefNum Registry Get.vi"("refnum name"="Chute 2") -> ("error out"=w284:errorcluster, "SolenoidDevRef"=w283:T6)  [unwired: 9 in]
          n147 = call <vilib>:"WPI_SolenoidRefNum Registry Get.vi"("refnum name"="Chute 1") -> ("error out"=w280:errorcluster, "SolenoidDevRef"=w279:T6)  [unwired: 9 in]
          n148 = call-poly <vilib>:"WPI_SolenoidSet.vi"("error in (no error)"=w284, "Value"=WPI_SolenoidValue."Off", "SolenoidDevRef"=w283) -> ()  [unwired: 7 in, 2 out]
          n149 = call-poly <vilib>:"WPI_SolenoidSet.vi"("error in (no error)"=w280, "Value"=WPI_SolenoidValue."On", "SolenoidDevRef"=w279) -> ()  [unwired: 7 in, 2 out]
        }
      }
    }
    frame "5" {
      # "Middle + Base Line Ft. Alan"
      n150 = flat-sequence {
        frame #0 {
          n151 = call <vilib>:"WPI_SolenoidRefNum Registry Get.vi"("refnum name"="Chute 2") -> ("error out"=w292:errorcluster, "SolenoidDevRef"=w291:T6)  [unwired: 9 in]
          n152 = call <vilib>:"WPI_SolenoidRefNum Registry Get.vi"("refnum name"="Chute 1") -> ("error out"=w288:errorcluster, "SolenoidDevRef"=w287:T6)  [unwired: 9 in]
          n153 = call-poly <vilib>:"WPI_SolenoidSet.vi"("error in (no error)"=w292, "Value"=WPI_SolenoidValue."On", "SolenoidDevRef"=w291) -> ()  [unwired: 7 in, 2 out]
          n154 = call-poly <vilib>:"WPI_SolenoidSet.vi"("error in (no error)"=w288, "Value"=WPI_SolenoidValue."Off", "SolenoidDevRef"=w287) -> ()  [unwired: 7 in, 2 out]
        }
        frame #1 {
          n155 = while {
            stop <- w300 stop-if-true
            n156 = call <vilib>:"WPI_RobotDriveRefNum Registry Get.vi"("refnum name"="Drive") -> ("error out"=w313:errorcluster, "RobotDriveDevRef"=w314:T8)  [unwired: 9 in]
            n157 = call <vilib>:"WPI_RobotDriveTankDrive.vi"("error in (no error)"=w313, "Right axis value"=-0.6323, "Left axis value"=-0.66, "RobotDriveDevRef"=w314) -> ()  [unwired: 5 in, 3 out]
            n158 = call <vilib>:"WPI_EncoderRefNum Registry Get.vi"("refnum name"="Encoder 0") -> ("error out"=w309:errorcluster, "EncoderDevRef"=w308:T13)  [unwired: 9 in]
            n159 = call <vilib>:"WPI_EncoderRefNum Registry Get.vi"("refnum name"="Encoder 1") -> ("error out"=w306:errorcluster, "EncoderDevRef"=w305:T13)  [unwired: 9 in]
            n160 = call <vilib>:"WPI_EncoderGet.vi"("error in (no error)"=w309, "EncoderDevRef"=w308) -> ("Distance"=w294:dbl)  [unwired: 4 in, 5 out]
            "Distance 6" <- w294
            n161 = Multiply(x=w294, y=-1.0) -> (x*y=w293:dbl)
            n162 = call <vilib>:"WPI_EncoderGet.vi"("error in (no error)"=w306, "EncoderDevRef"=w305) -> ("Distance"=w297:dbl)  [unwired: 4 in, 5 out]
            "Distance 7" <- w297
            n163 = Add(x=w293, y=w297) -> (x+y=w303:dbl)
            n164 = call-poly <vilib>:"NT Write Value.vi"("Numeric"=w294, "Name"="Encoder 0") -> ()  [unwired: 9 in, 1 out]
            n165 = call-poly <vilib>:"NT Write Value.vi"("Numeric"=w297, "Name"="Encoder 1") -> ()  [unwired: 9 in, 1 out]
            n166 = Divide(x=w303, y=2.0) -> (x/y=w301:dbl)
            n167 = Less?(x=w301, y=-0.68) -> (x < y?=w300:bool)
          }
        }
        frame #2 {
          n168 = call <vilib>:"WPI_RobotDriveRefNum Registry Get.vi"("refnum name"="Drive") -> ("error out"=w318:errorcluster, "RobotDriveDevRef"=w319:T8)  [unwired: 9 in]
          n169 = call <vilib>:"WPI_RobotDriveTankDrive.vi"("error in (no error)"=w318, "Right axis value"=0.0, "Left axis value"=0.0, "RobotDriveDevRef"=w319) -> ("error out"=w321:errorcluster, "RobotDriveDevRef"=w320:T8)  [unwired: 5 in, 1 out]
          n170 = call <vilib>:"WPI_RobotDriveDelayAndUpdateSafety.vi"("error in (no error)"=w321, "Delay (s)"=2.0, "RobotDriveDevRef"=w320) -> ()  [unwired: 7 in, 2 out]
        }
        frame #3 {
          n171 = call <vilib>:"WPI_SolenoidRefNum Registry Get.vi"("refnum name"="Chute 2") -> ("error out"=w330:errorcluster, "SolenoidDevRef"=w329:T6)  [unwired: 9 in]
          n172 = call <vilib>:"WPI_SolenoidRefNum Registry Get.vi"("refnum name"="Chute 1") -> ("error out"=w326:errorcluster, "SolenoidDevRef"=w325:T6)  [unwired: 9 in]
          n173 = call-poly <vilib>:"WPI_SolenoidSet.vi"("error in (no error)"=w330, "Value"=WPI_SolenoidValue."Off", "SolenoidDevRef"=w329) -> ()  [unwired: 7 in, 2 out]
          n174 = call-poly <vilib>:"WPI_SolenoidSet.vi"("error in (no error)"=w326, "Value"=WPI_SolenoidValue."On", "SolenoidDevRef"=w325) -> ()  [unwired: 7 in, 2 out]
        }
        frame #4 {
          n175 = call <vilib>:"WPI_RobotDriveRefNum Registry Get.vi"("refnum name"="Drive") -> ("error out"=w334:errorcluster, "RobotDriveDevRef"=w335:T8)  [unwired: 9 in]
          n176 = call <vilib>:"WPI_RobotDriveTankDrive.vi"("error in (no error)"=w334, "Right axis value"=0.0, "Left axis value"=0.0, "RobotDriveDevRef"=w335) -> ("error out"=w337:errorcluster, "RobotDriveDevRef"=w336:T8)  [unwired: 5 in, 1 out]
          n177 = call <vilib>:"WPI_RobotDriveDelayAndUpdateSafety.vi"("error in (no error)"=w337, "Delay (s)"=2.0, "RobotDriveDevRef"=w336) -> ()  [unwired: 7 in, 2 out]
        }
      }
    }
    frame "6" {
      # "Left Peg"
      n178 = flat-sequence {
        frame #0 {
          n179 = call <vilib>:"WPI_SolenoidRefNum Registry Get.vi"("refnum name"="Chute 2") -> ("error out"=w346:errorcluster, "SolenoidDevRef"=w345:T6)  [unwired: 9 in]
          n180 = call <vilib>:"WPI_SolenoidRefNum Registry Get.vi"("refnum name"="Chute 1") -> ("error out"=w342:errorcluster, "SolenoidDevRef"=w341:T6)  [unwired: 9 in]
          n181 = call-poly <vilib>:"WPI_SolenoidSet.vi"("error in (no error)"=w346, "Value"=WPI_SolenoidValue."On", "SolenoidDevRef"=w345) -> ()  [unwired: 7 in, 2 out]
          n182 = call-poly <vilib>:"WPI_SolenoidSet.vi"("error in (no error)"=w342, "Value"=WPI_SolenoidValue."Off", "SolenoidDevRef"=w341) -> ()  [unwired: 7 in, 2 out]
        }
        frame #1 {
          n183 = while {
            stop <- w354 stop-if-true
            n184 = call <vilib>:"WPI_RobotDriveRefNum Registry Get.vi"("refnum name"="Drive") -> ("error out"=w367:errorcluster, "RobotDriveDevRef"=w368:T8)  [unwired: 9 in]
            n185 = call <vilib>:"WPI_RobotDriveTankDrive.vi"("error in (no error)"=w367, "Right axis value"=-0.6323, "Left axis value"=-0.66, "RobotDriveDevRef"=w368) -> ()  [unwired: 5 in, 3 out]
            n186 = call <vilib>:"WPI_EncoderRefNum Registry Get.vi"("refnum name"="Encoder 0") -> ("error out"=w363:errorcluster, "EncoderDevRef"=w362:T13)  [unwired: 9 in]
            n187 = call <vilib>:"WPI_EncoderRefNum Registry Get.vi"("refnum name"="Encoder 1") -> ("error out"=w360:errorcluster, "EncoderDevRef"=w359:T13)  [unwired: 9 in]
            n188 = call <vilib>:"WPI_EncoderGet.vi"("error in (no error)"=w363, "EncoderDevRef"=w362) -> ("Distance"=w348:dbl)  [unwired: 4 in, 5 out]
            "Distance 8" <- w348
            n189 = Multiply(x=w348, y=-1.0) -> (x*y=w347:dbl)
            n190 = call <vilib>:"WPI_EncoderGet.vi"("error in (no error)"=w360, "EncoderDevRef"=w359) -> ("Distance"=w351:dbl)  [unwired: 4 in, 5 out]
            "Distance 9" <- w351
            n191 = Add(x=w347, y=w351) -> (x+y=w357:dbl)
            n192 = call-poly <vilib>:"NT Write Value.vi"("Numeric"=w348, "Name"="Encoder 0") -> ()  [unwired: 9 in, 1 out]
            n193 = call-poly <vilib>:"NT Write Value.vi"("Numeric"=w351, "Name"="Encoder 1") -> ()  [unwired: 9 in, 1 out]
            n194 = Divide(x=w357, y=2.0) -> (x/y=w355:dbl)
            n195 = Less?(x=w355, y=-0.68) -> (x < y?=w354:bool)
          }
        }
        frame #2 {
          n196 = call <vilib>:"WPI_RobotDriveRefNum Registry Get.vi"("refnum name"="Drive") -> ("error out"=w372:errorcluster, "RobotDriveDevRef"=w373:T8)  [unwired: 9 in]
          n197 = call <vilib>:"WPI_RobotDriveTankDrive.vi"("error in (no error)"=w372, "Right axis value"=0.0, "Left axis value"=0.0, "RobotDriveDevRef"=w373) -> ("error out"=w375:errorcluster, "RobotDriveDevRef"=w374:T8)  [unwired: 5 in, 1 out]
          n198 = call <vilib>:"WPI_RobotDriveDelayAndUpdateSafety.vi"("error in (no error)"=w375, "Delay (s)"=2.0, "RobotDriveDevRef"=w374) -> ()  [unwired: 7 in, 2 out]
        }
        frame #3 {
          n199 = call <vilib>:"WPI_RobotDriveRefNum Registry Get.vi"("refnum name"="Drive") -> ("error out"=w381:errorcluster, "RobotDriveDevRef"=w380:T8)  [unwired: 9 in]
          n200 = call <vilib>:"WPI_RobotDriveTankDrive.vi"("error in (no error)"=w381, "Right axis value"=0.6, "Left axis value"=-0.6, "RobotDriveDevRef"=w380) -> ("error out"=w378:errorcluster, "RobotDriveDevRef"=w379:T8)  [unwired: 5 in, 1 out]
          n201 = call <vilib>:"WPI_RobotDriveDelayAndUpdateSafety.vi"("error in (no error)"=w378, "Delay (s)"=1.0, "RobotDriveDevRef"=w379) -> ()  [unwired: 7 in, 2 out]
        }
        frame #4 {
          n202 = call <vilib>:"WPI_RobotDriveRefNum Registry Get.vi"("refnum name"="Drive") -> ("error out"=w389:errorcluster, "RobotDriveDevRef"=w388:T8)  [unwired: 9 in]
          n203 = call <vilib>:"WPI_RobotDriveTankDrive.vi"("error in (no error)"=w389, "Right axis value"=-0.5, "Left axis value"=-0.5, "RobotDriveDevRef"=w388) -> ("error out"=w386:errorcluster, "RobotDriveDevRef"=w387:T8)  [unwired: 5 in, 1 out]
          n204 = call <vilib>:"WPI_RobotDriveDelayAndUpdateSafety.vi"("error in (no error)"=w386, "Delay (s)"=2.0, "RobotDriveDevRef"=w387) -> ()  [unwired: 7 in, 2 out]
        }
        frame #5 {
          n205 = call <vilib>:"WPI_SolenoidRefNum Registry Get.vi"("refnum name"="Chute 2") -> ("error out"=w400:errorcluster, "SolenoidDevRef"=w399:T6)  [unwired: 9 in]
          n206 = call <vilib>:"WPI_SolenoidRefNum Registry Get.vi"("refnum name"="Chute 1") -> ("error out"=w396:errorcluster, "SolenoidDevRef"=w395:T6)  [unwired: 9 in]
          n207 = call-poly <vilib>:"WPI_SolenoidSet.vi"("error in (no error)"=w400, "Value"=WPI_SolenoidValue."Off", "SolenoidDevRef"=w399) -> ()  [unwired: 7 in, 2 out]
          n208 = call-poly <vilib>:"WPI_SolenoidSet.vi"("error in (no error)"=w396, "Value"=WPI_SolenoidValue."On", "SolenoidDevRef"=w395) -> ()  [unwired: 7 in, 2 out]
        }
        frame #6 {
          n209 = call <vilib>:"WPI_RobotDriveRefNum Registry Get.vi"("refnum name"="Drive") -> ("error out"=w404:errorcluster, "RobotDriveDevRef"=w405:T8)  [unwired: 9 in]
          n210 = call <vilib>:"WPI_RobotDriveTankDrive.vi"("error in (no error)"=w404, "Right axis value"=0.0, "Left axis value"=0.0, "RobotDriveDevRef"=w405) -> ("error out"=w407:errorcluster, "RobotDriveDevRef"=w406:T8)  [unwired: 5 in, 1 out]
          n211 = call <vilib>:"WPI_RobotDriveDelayAndUpdateSafety.vi"("error in (no error)"=w407, "Delay (s)"=1.0, "RobotDriveDevRef"=w406) -> ()  [unwired: 7 in, 2 out]
        }
        frame #7 {
          n212 = call <vilib>:"WPI_RobotDriveRefNum Registry Get.vi"("refnum name"="Drive") -> ("error out"=w413:errorcluster, "RobotDriveDevRef"=w412:T8)  [unwired: 9 in]
          n213 = call <vilib>:"WPI_RobotDriveTankDrive.vi"("error in (no error)"=w413, "Right axis value"=0.5, "Left axis value"=0.5, "RobotDriveDevRef"=w412) -> ("error out"=w410:errorcluster, "RobotDriveDevRef"=w411:T8)  [unwired: 5 in, 1 out]
          n214 = call <vilib>:"WPI_RobotDriveDelayAndUpdateSafety.vi"("error in (no error)"=w410, "Delay (s)"=1.5, "RobotDriveDevRef"=w411) -> ()  [unwired: 7 in, 2 out]
        }
      }
    }
    frame "7" {
      n215 = flat-sequence {
        frame #0 {
          n216 = call <vilib>:"WPI_SolenoidRefNum Registry Get.vi"("refnum name"="Chute 2") -> ("error out"=w424:errorcluster, "SolenoidDevRef"=w423:T6)  [unwired: 9 in]
          n217 = call <vilib>:"WPI_SolenoidRefNum Registry Get.vi"("refnum name"="Chute 1") -> ("error out"=w420:errorcluster, "SolenoidDevRef"=w419:T6)  [unwired: 9 in]
          n218 = call-poly <vilib>:"WPI_SolenoidSet.vi"("error in (no error)"=w424, "Value"=WPI_SolenoidValue."On", "SolenoidDevRef"=w423) -> ()  [unwired: 7 in, 2 out]
          n219 = call-poly <vilib>:"WPI_SolenoidSet.vi"("error in (no error)"=w420, "Value"=WPI_SolenoidValue."Off", "SolenoidDevRef"=w419) -> ()  [unwired: 7 in, 2 out]
        }
        frame #1 {
          n220 = while {
            stop <- w432 stop-if-true
            n221 = call <vilib>:"WPI_RobotDriveRefNum Registry Get.vi"("refnum name"="Drive") -> ("error out"=w445:errorcluster, "RobotDriveDevRef"=w446:T8)  [unwired: 9 in]
            n222 = call <vilib>:"WPI_RobotDriveTankDrive.vi"("error in (no error)"=w445, "Right axis value"=-0.6323, "Left axis value"=-0.66, "RobotDriveDevRef"=w446) -> ()  [unwired: 5 in, 3 out]
            n223 = call <vilib>:"WPI_EncoderRefNum Registry Get.vi"("refnum name"="Encoder 0") -> ("error out"=w441:errorcluster, "EncoderDevRef"=w440:T13)  [unwired: 9 in]
            n224 = call <vilib>:"WPI_EncoderRefNum Registry Get.vi"("refnum name"="Encoder 1") -> ("error out"=w438:errorcluster, "EncoderDevRef"=w437:T13)  [unwired: 9 in]
            n225 = call <vilib>:"WPI_EncoderGet.vi"("error in (no error)"=w441, "EncoderDevRef"=w440) -> ("Distance"=w426:dbl)  [unwired: 4 in, 5 out]
            "Distance 10" <- w426
            n226 = Multiply(x=w426, y=-1.0) -> (x*y=w425:dbl)
            n227 = call <vilib>:"WPI_EncoderGet.vi"("error in (no error)"=w438, "EncoderDevRef"=w437) -> ("Distance"=w429:dbl)  [unwired: 4 in, 5 out]
            "Distance 11" <- w429
            n228 = Add(x=w425, y=w429) -> (x+y=w435:dbl)
            n229 = call-poly <vilib>:"NT Write Value.vi"("Numeric"=w426, "Name"="Encoder 0") -> ()  [unwired: 9 in, 1 out]
            n230 = call-poly <vilib>:"NT Write Value.vi"("Numeric"=w429, "Name"="Encoder 1") -> ()  [unwired: 9 in, 1 out]
            n231 = Divide(x=w435, y=2.0) -> (x/y=w433:dbl)
            n232 = Less?(x=w433, y=-0.78) -> (x < y?=w432:bool)
          }
        }
        frame #2 {
          n233 = call <vilib>:"WPI_RobotDriveRefNum Registry Get.vi"("refnum name"="Drive") -> ("error out"=w450:errorcluster, "RobotDriveDevRef"=w451:T8)  [unwired: 9 in]
          n234 = call <vilib>:"WPI_RobotDriveTankDrive.vi"("error in (no error)"=w450, "Right axis value"=0.0, "Left axis value"=0.0, "RobotDriveDevRef"=w451) -> ("error out"=w453:errorcluster, "RobotDriveDevRef"=w452:T8)  [unwired: 5 in, 1 out]
          n235 = call <vilib>:"WPI_RobotDriveDelayAndUpdateSafety.vi"("error in (no error)"=w453, "Delay (s)"=2.0, "RobotDriveDevRef"=w452) -> ()  [unwired: 7 in, 2 out]
        }
        frame #3 {
          n236 = call <vilib>:"WPI_RobotDriveRefNum Registry Get.vi"("refnum name"="Drive") -> ("error out"=w459:errorcluster, "RobotDriveDevRef"=w458:T8)  [unwired: 9 in]
          n237 = call <vilib>:"WPI_RobotDriveTankDrive.vi"("error in (no error)"=w459, "Right axis value"=-0.6, "Left axis value"=0.6, "RobotDriveDevRef"=w458) -> ("error out"=w456:errorcluster, "RobotDriveDevRef"=w457:T8)  [unwired: 5 in, 1 out]
          n238 = call <vilib>:"WPI_RobotDriveDelayAndUpdateSafety.vi"("error in (no error)"=w456, "Delay (s)"=0.8, "RobotDriveDevRef"=w457) -> ()  [unwired: 7 in, 2 out]
        }
        frame #4 {
          n239 = call <vilib>:"WPI_RobotDriveRefNum Registry Get.vi"("refnum name"="Drive") -> ("error out"=w467:errorcluster, "RobotDriveDevRef"=w466:T8)  [unwired: 9 in]
          n240 = call <vilib>:"WPI_RobotDriveTankDrive.vi"("error in (no error)"=w467, "Right axis value"=-0.5, "Left axis value"=-0.5, "RobotDriveDevRef"=w466) -> ("error out"=w464:errorcluster, "RobotDriveDevRef"=w465:T8)  [unwired: 5 in, 1 out]
          n241 = call <vilib>:"WPI_RobotDriveDelayAndUpdateSafety.vi"("error in (no error)"=w464, "Delay (s)"=1.8, "RobotDriveDevRef"=w465) -> ()  [unwired: 7 in, 2 out]
        }
        frame #5 {
          n242 = call <vilib>:"WPI_SolenoidRefNum Registry Get.vi"("refnum name"="Chute 2") -> ("error out"=w478:errorcluster, "SolenoidDevRef"=w477:T6)  [unwired: 9 in]
          n243 = call <vilib>:"WPI_SolenoidRefNum Registry Get.vi"("refnum name"="Chute 1") -> ("error out"=w474:errorcluster, "SolenoidDevRef"=w473:T6)  [unwired: 9 in]
          n244 = call-poly <vilib>:"WPI_SolenoidSet.vi"("error in (no error)"=w478, "Value"=WPI_SolenoidValue."Off", "SolenoidDevRef"=w477) -> ()  [unwired: 7 in, 2 out]
          n245 = call-poly <vilib>:"WPI_SolenoidSet.vi"("error in (no error)"=w474, "Value"=WPI_SolenoidValue."On", "SolenoidDevRef"=w473) -> ()  [unwired: 7 in, 2 out]
        }
        frame #6 {
          n246 = call <vilib>:"WPI_RobotDriveRefNum Registry Get.vi"("refnum name"="Drive") -> ("error out"=w482:errorcluster, "RobotDriveDevRef"=w483:T8)  [unwired: 9 in]
          n247 = call <vilib>:"WPI_RobotDriveTankDrive.vi"("error in (no error)"=w482, "Right axis value"=0.0, "Left axis value"=0.0, "RobotDriveDevRef"=w483) -> ("error out"=w485:errorcluster, "RobotDriveDevRef"=w484:T8)  [unwired: 5 in, 1 out]
          n248 = call <vilib>:"WPI_RobotDriveDelayAndUpdateSafety.vi"("error in (no error)"=w485, "Delay (s)"=1.0, "RobotDriveDevRef"=w484) -> ()  [unwired: 7 in, 2 out]
        }
        frame #7 {
          n249 = call <vilib>:"WPI_RobotDriveRefNum Registry Get.vi"("refnum name"="Drive") -> ("error out"=w491:errorcluster, "RobotDriveDevRef"=w490:T8)  [unwired: 9 in]
          n250 = call <vilib>:"WPI_RobotDriveTankDrive.vi"("error in (no error)"=w491, "Right axis value"=0.5, "Left axis value"=0.5, "RobotDriveDevRef"=w490) -> ("error out"=w488:errorcluster, "RobotDriveDevRef"=w489:T8)  [unwired: 5 in, 1 out]
          n251 = call <vilib>:"WPI_RobotDriveDelayAndUpdateSafety.vi"("error in (no error)"=w488, "Delay (s)"=1.5, "RobotDriveDevRef"=w489) -> ()  [unwired: 7 in, 2 out]
        }
      }
    }
  }
